vi "file or path.vi"(2 "Path":path=path "Faraday Cup Control System.xml") -> (0 "file/path&file":bool)   [LabVIEW 2013, in "OPCUA XML.lvlib"]
uses:
  OPCUA XML.lvlib
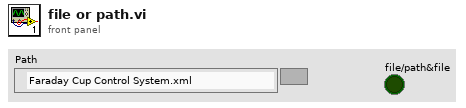
[diagram p1: front panel]
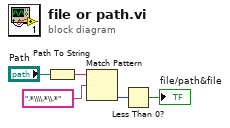
[diagram p0: block diagram]
diagram:
  n1 = Path To String(path="Path") -> (string=w4:string)
  n2 = Match Pattern(string=w4, regular expression=".*\\\\.*\\.*") -> (offset past match=w2:i32)  [unwired: 1 in, 3 out]
  n3 = Less Than 0?(x=w2) -> (x < 0?=→"file/path&file":bool)
